vi "Generic_Cross_Moments.vi"(2 "Cluster2":T1={"Colour"=0, "Inst type"=enum."Pitot-static tube", "Inst name"="Manometer voltage", "Symbol"="U", "Code name"="", "Extra Info"="U", "Inst Array"=enum."PWA", "Index"=0, "Voltage Index"=0, "Extra Titles"=[], "Extra Values"=[], "Eng Values"=[], "Time (ms)"=[], "TT / Voltage"=[], "u^2"=0.0, "U"=0.0, "u^3/(u^2)^(1.5)"=0.0, "u^4"=0.0, "u^4/(u^2)^2 -3"=0.0, "Mean % Err"=0.0, "% u'/U"=0.0} {"% u'/U" format="%.2f"; "Mean % Err" format="%.2f"; "u^4/(u^2)^2 -3" format="%.2f"; "u^4" format="%.2f"; "u^3/(u^2)^(1.5)" format="%.2f"; "U" format="%.2f"; "u^2" format="%.2f"}, 3 "Cluster1":T1={"Colour"=0, "Inst type"=enum."Pitot-static tube", "Inst name"="Manometer voltage", "Symbol"="U", "Code name"="", "Extra Info"="U", "Inst Array"=enum."PWA", "Index"=0, "Voltage Index"=0, "Extra Titles"=[], "Extra Values"=[], "Eng Values"=[], "Time (ms)"=[], "TT / Voltage"=[], "u^2"=0.0, "U"=0.0, "u^3/(u^2)^(1.5)"=0.0, "u^4"=0.0, "u^4/(u^2)^2 -3"=0.0, "Mean % Err"=0.0, "% u'/U"=0.0} {"% u'/U" format="%.2f"; "Mean % Err" format="%.2f"; "u^4/(u^2)^2 -3" format="%.2f"; "u^4" format="%.2f"; "u^3/(u^2)^(1.5)" format="%.2f"; "U" format="%.2f"; "u^2" format="%.2f"}) -> (0 "Plug in Values":dbl[](array[numeric]), 1 "Plug in titles":string[](array[string]))   [LabVIEW 2011]
uses:
  Controls/Analysis_info_cluster.ctl
  Controls/Inst_type.ctl
  Controls/Instrument_Array.ctl
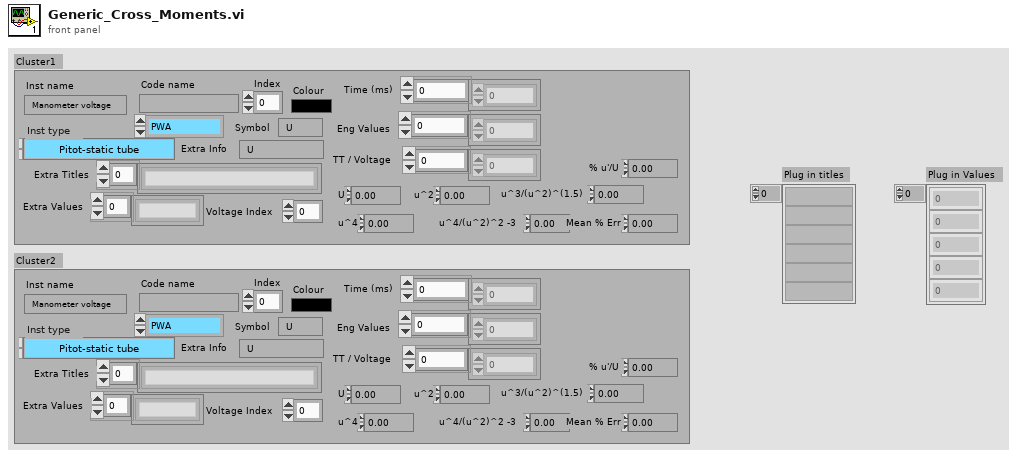
[diagram p1: front panel]
types:
  T1 = typedef "Analysis_info_cluster.ctl" = cluster{"Colour":u32, "Inst type":T2, "Inst name":string, "Symbol":string, "Code name":string, "Extra Info":string, "Inst Array":T3, "Index":i32, "Voltage Index":i32, "Extra Titles":string[], "Extra Values":string[], "Eng Values":dbl[], "Time (ms)":dbl[], "TT / Voltage":dbl[], "u^2":dbl, "U":dbl, "u^3/(u^2)^(1.5)":dbl, "u^4":dbl, "u^4/(u^2)^2 -3":dbl, "Mean % Err":dbl, "% u'/U":dbl}
  T2 = typedef "Inst_type.ctl" = enum16{"Propeller anemometer", "Raw voltage", "Pressure Transducer", "Pitot-static tube", "Preston tube", "Hot wire", "Cross wire 1", "Cross wire 2", "Generic Linear", "Generic Polynomial", "Generic BackPoly", "Fast FID", "Thermocouple", "Cold wire", "Pulsed Wire", "LDA Vel", "LDA Tran time", "LDA Arr time"}
  T3 = typedef "Instrument_Array.ctl" = enum16{"PWA", "LDA", "Analogue"}
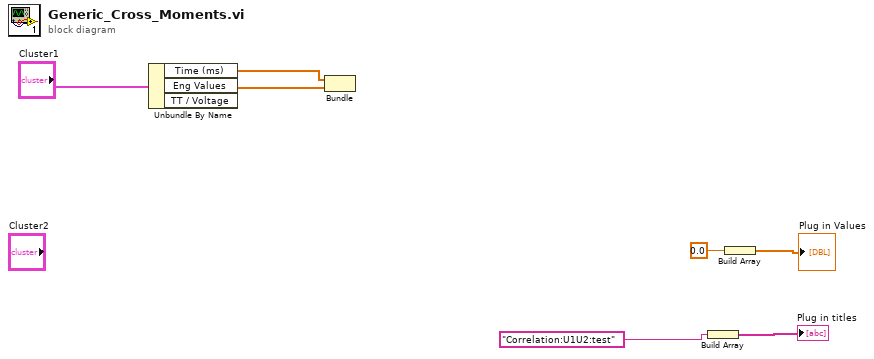
[diagram p0: block diagram]
diagram:
  n1 = Unbundle By Name("Cluster1") -> ("Time (ms)"=w2:dbl[], "Eng Values"=w3:dbl[])  [unwired: 1 out]
  n2 = Bundle("Time (ms)"=w2, "Eng Values"=w3) -> ()  [unwired: 1 in, 1 out]
  n3 = Build Array("Correlation:U1U2:test") -> (→"Plug in titles":string[])
  n4 = Build Array(0.0 ("Numeric")) -> (→"Plug in Values":dbl[])
